vi "Run Contest.vi"() -> ()   [LabVIEW 2014]
uses:
  Participant.ctl
  Problem.ctl
  State Machine.ctl
  User Score Update.ctl
  Change Detect/Change Detect Int.vi
  Change Detect/Change Detect Boolean.vi
panel:
  in  "Update Ratings":bool
  in  "Early Finish":bool
  in  "Export Results":bool
  in  "Participant Names":string[](array[string])
  in  "Contest Length (hours)":dbl
  in  "Problem E Base Value":dbl=2500.0
  in  "Problem D Base Value":dbl=2000.0
  in  "Problem C Base Value":dbl=1500.0
  in  "Problem B Base Value":dbl=1000.0
  in  "Problem A Base Value":dbl=500.0
  in  "OK Button":bool
  in  "Problem":T1
  in  "Participant":string
  in  "At Time Remaining":dbl=3600.0
  out "Participant Status":T2[](array[typedef])
  in  "Participants":dbl
  in  "Contest Start":bool
  out "Time Remaining":u32
  out "Contest Indicator":bool
  out "Problem E Current Value":dbl
  out "Problem D Current Value":dbl
  out "Problem C Current Value":dbl
  out "Problem B Current Value":dbl
  out "Problem A Current Value":dbl
  # "You must export before starting a new Contest"
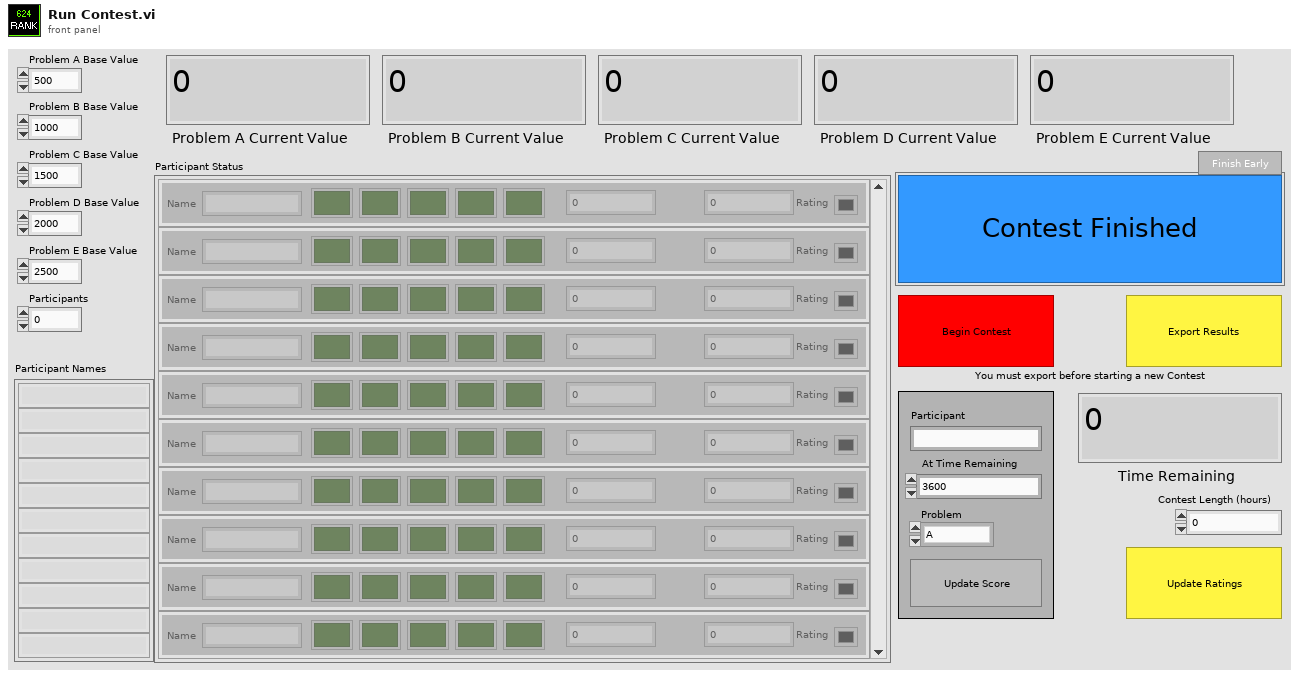
[diagram p1: front panel]
types:
  T1 = typedef "Problem.ctl" = enum16{"A", "B", "C", "D", "E"}
  T2 = typedef "Participant.ctl" = cluster{"Name":string, "A":bool, "Score":dbl, "B":bool, "C":bool, "D":bool, "E":bool, "Rating":dbl, "Color Box":u32}
  T3 = typedef "State Machine.ctl" = enum16{"Finish Contest", "Run Contest", "Begin Contest", "Wait for Start"}
  T4 = typedef "User Score Update.ctl" = cluster{"Score":dbl, "Name":string}
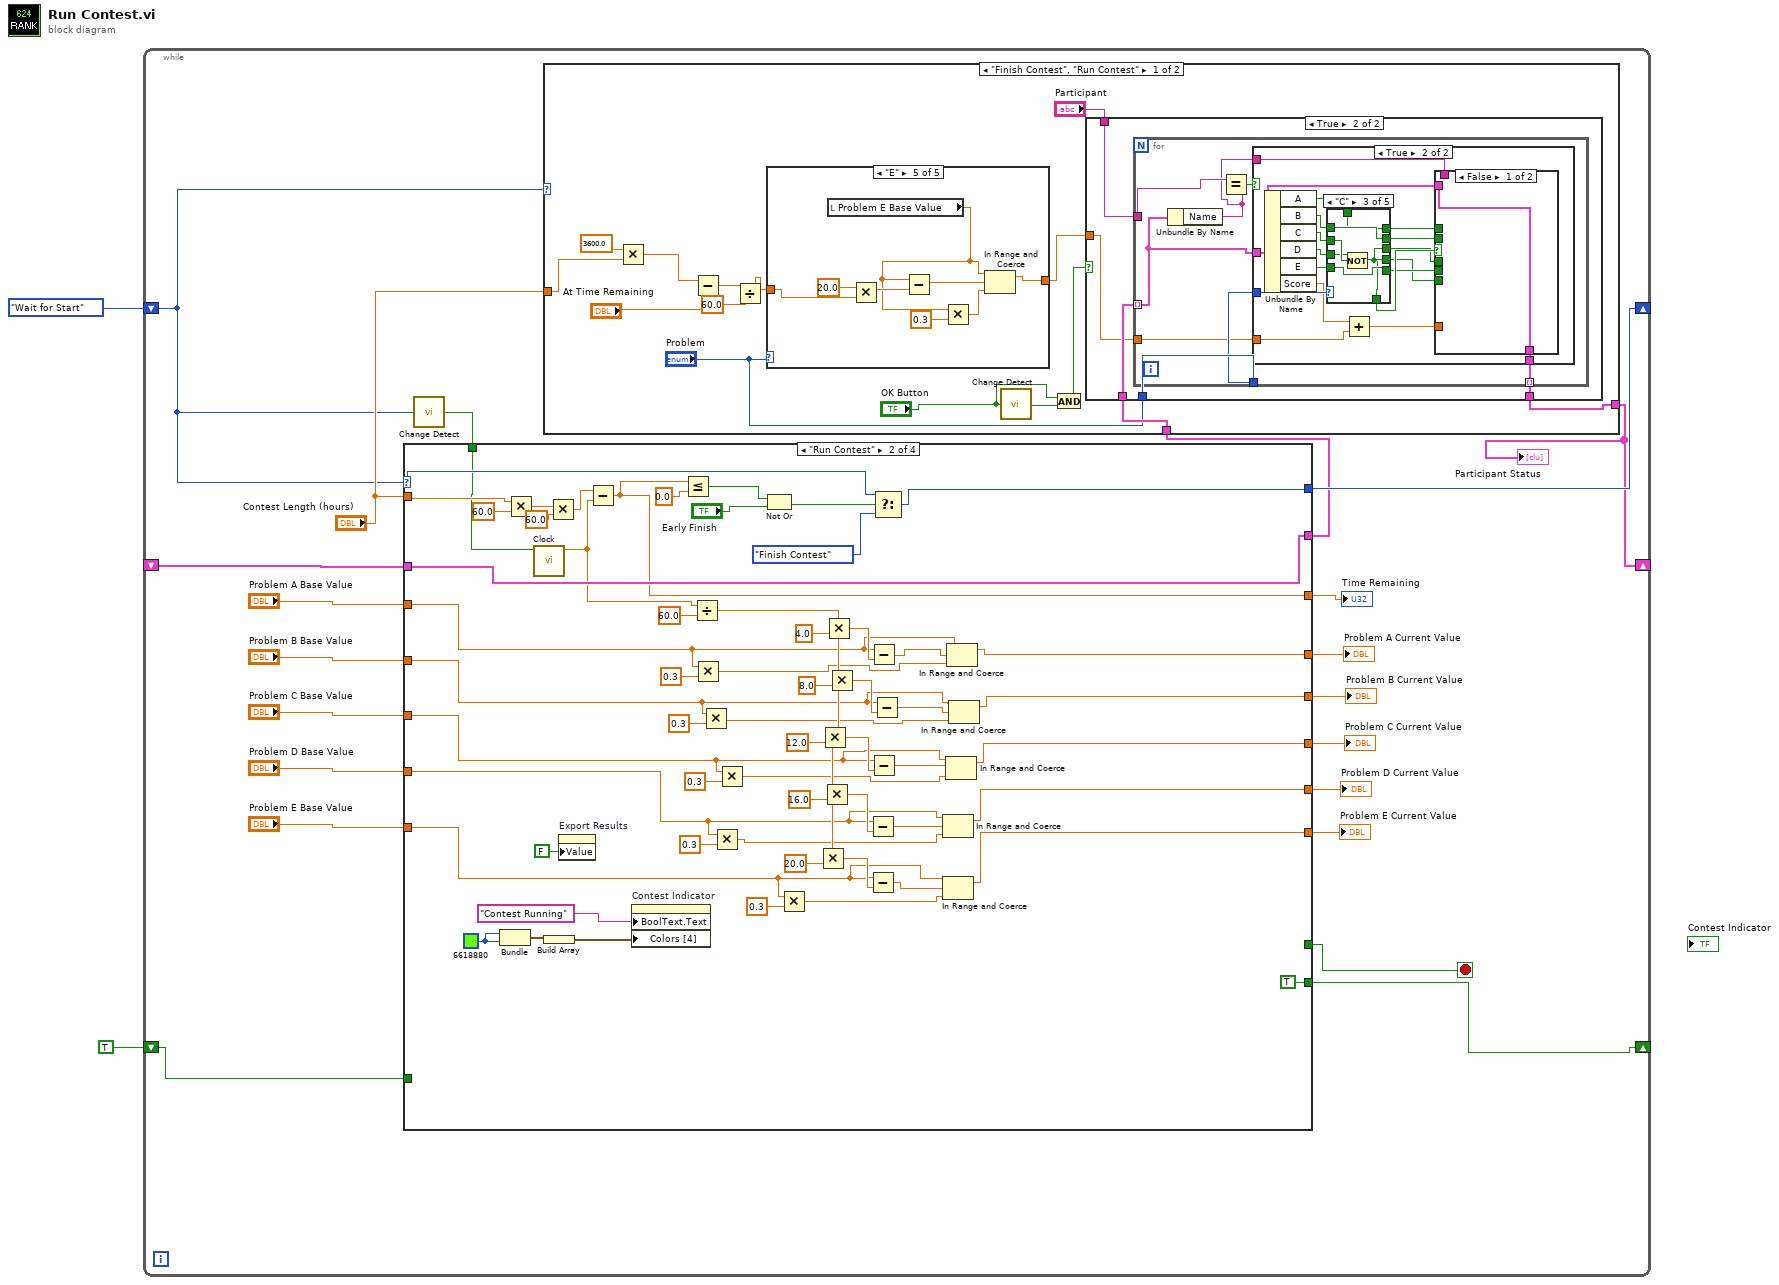
[diagram p0: block diagram]
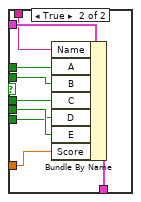
[diagram p4: hidden frame]
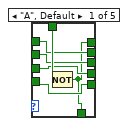
[diagram p5: hidden frame]
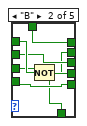
[diagram p6: hidden frame]
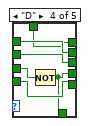
[diagram p7: hidden frame]
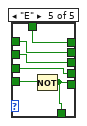
[diagram p8: hidden frame]
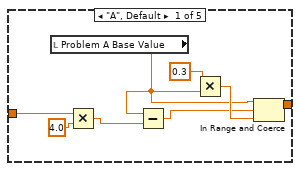
[diagram p9: hidden frame]
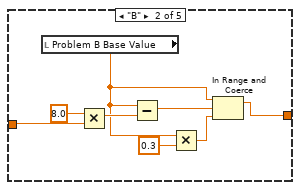
[diagram p10: hidden frame]
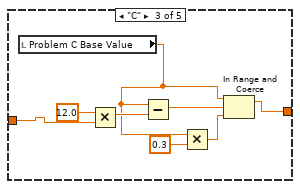
[diagram p11: hidden frame]
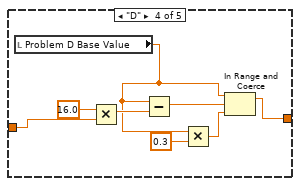
[diagram p12: hidden frame]
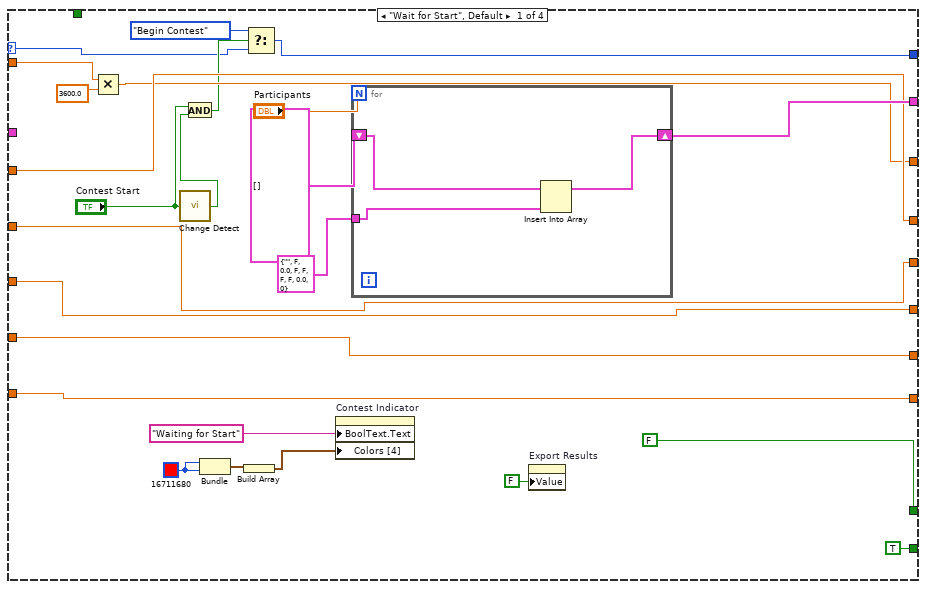
[diagram p14: hidden frame]
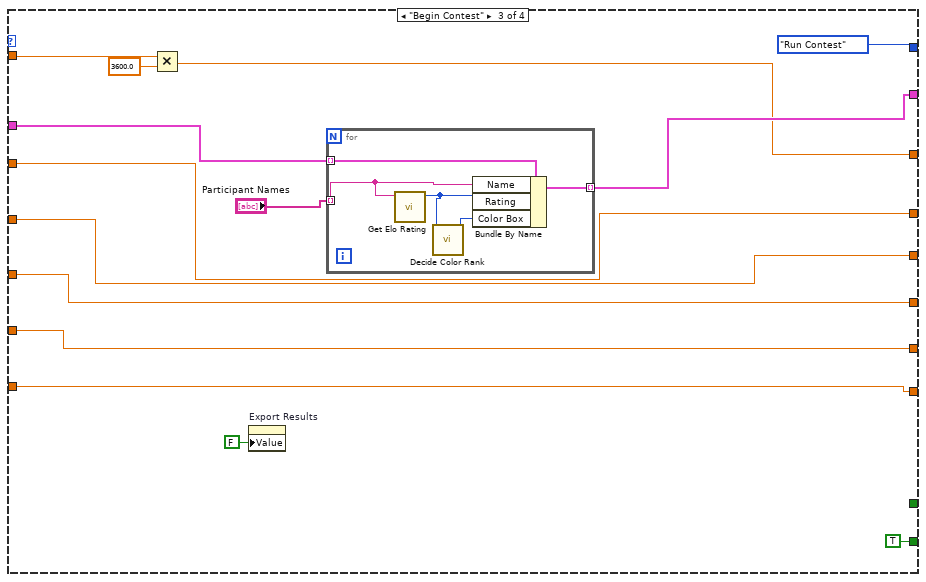
[diagram p15: hidden frame]
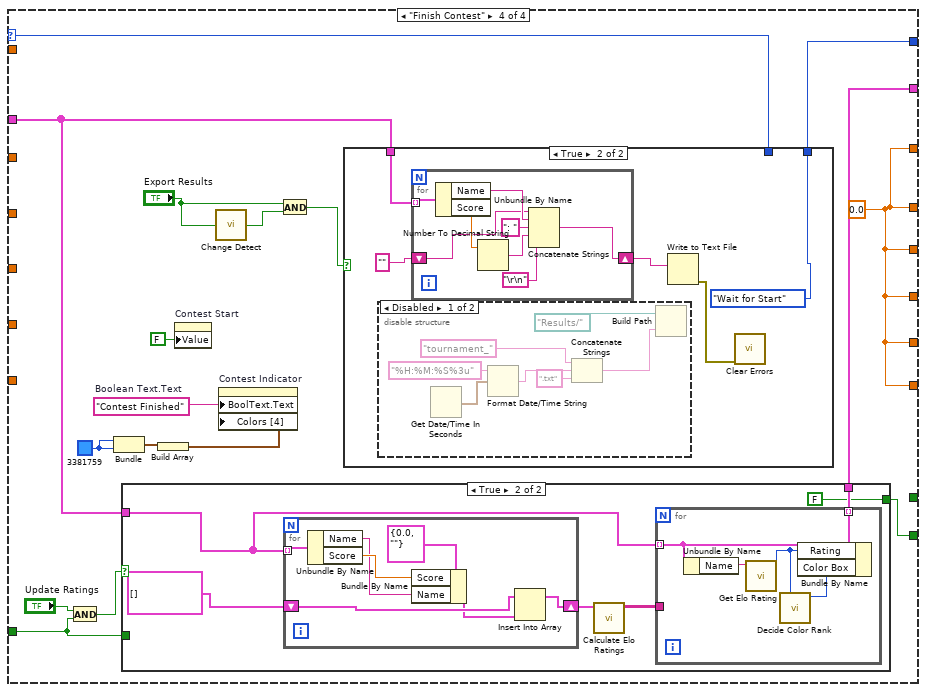
[diagram p16: hidden frame]
diagram:
  n1 = while {
    shift-right: [w6] -> _
    shift-left: _ -> [w22]
    shift-right: [w16] -> _
    shift-left: State_Machine."Wait for Start" -> [w5]
    shift-right: [w3] -> _
    shift-left: TRUE -> [w4]
    stop <- w23 stop-if-true
    n2 = call-poly "Change Detect.vi"("In"=w5) -> ("Changed?"=w9:bool)
    n3 = case shown="\"Run Contest\"" w5 {
      selector: w5 -> [w154 w228 _ w266]
      tunnel: [FALSE _ _ _] -> w23
      tunnel: [w172 w226 w250 w262] -> w7
      tunnel: w22 -> [_ w226 w251 w263]
      tunnel: "Problem A Base Value" -> [w163 w211 w248 _]
      tunnel: "Problem B Base Value" -> [w164 w203 w247 _]
      tunnel: "Problem C Base Value" -> [w165 w200 w246 _]
      tunnel: "Problem D Base Value" -> [w166 w195 w245 _]
      tunnel: "Problem E Base Value" -> [w167 w192 w244 _]
      tunnel: "Contest Length (hours)" -> [w162 w230 w243 _]
      tunnel: [w153 w227 State_Machine."Run Contest" w265] -> w16
      tunnel: [w163 w212 w248 w270] -> w15
      tunnel: [w164 w201 w247 w270] -> w14
      tunnel: [w165 w197 w246 w270] -> w13
      tunnel: [w166 w193 w245 w270] -> w12
      tunnel: [w167 w189 w244 w270] -> w11
      tunnel: [w160 w188 w241 w270] -> w10
      tunnel: w9 -> [_ w187 _ _]
      tunnel: w4 -> [_ _ _ w258]
      tunnel: [TRUE TRUE TRUE w259] -> w3
      frame "Wait for Start", Default {
        w170 = u32 16711680
        n4 = Multiply(x=w162, y=3600.0) -> (x*y=w160:dbl)
        n5 = call-poly "Change Detect.vi"("In"="Contest Start") -> ("Changed?"=w157:bool)
        n6 = And(x="Contest Start", y=w157) -> (x .and. y?=w156:bool)
        n7 = Bundle(w170, w170) -> (w169:cluster{u32, u32})  [unwired: 1 in]
        n8 = Build Array(w169) -> (w168:cluster{u32, u32}[])
        n9 = Select(t=State_Machine."Begin Contest", s=w156, f=w154) -> (s? t:f=w153:T3)
        n10 = property on="Contest Indicator" class="Bool (strict)"("BoolText.Text"="Waiting for Start" ("Boolean Text.Text"), "Colors [4]"=w168) -> ()  [unwired: 2 in, 2 out]
        n11 = for {
          N: "Participants" -> [_]
          shift-right: [w179] -> w172
          shift-left: T2[] [] ("array") -> [w178]
          tunnel: T2 {"Name"="", "A"=FALSE, "Score"=0.0, "B"=FALSE, "C"=FALSE, "D"=FALSE, "E"=FALSE, "Rating"=0.0, "Color Box"=0} ("Participant") -> [w177]
          n12 = Insert Into Array(array=w178, new element=w177) -> (w179:T2[])  [unwired: 1 in]
        }
        n13 = property on="Export Results" class="Bool (strict)"("Value"=FALSE ("Export Results")) -> ()  [unwired: 2 in, 2 out]
      }
      frame "Run Contest" {
        w237 = u32 6618880
        n14 = Bundle(w237, w237) -> (w236:cluster{u32, u32})  [unwired: 1 in]
        n15 = Multiply(x=w230, y=60.0) -> (x*y=w232:dbl)
        n16 = call "Clock.vi"("Reset?"=w187) -> ("Time Elapsed"=w186:dbl)  [unwired: 10 in]
        n17 = Build Array(w236) -> (w235:cluster{u32, u32}[])
        n18 = Multiply(x=w232, y=60.0) -> (x*y=w234:dbl)
        n19 = property on="Export Results" class="Bool (strict)"("Value"=FALSE ("Export Results")) -> ()  [unwired: 2 in, 2 out]
        n20 = Subtract(x=w234, y=w186) -> (x-y=w188:dbl)
        n21 = property on="Contest Indicator" class="Bool (strict)"("BoolText.Text"="Contest Running" ("Boolean Text.Text"), "Colors [4]"=w235) -> ()  [unwired: 2 in, 2 out]
        n22 = Less Or Equal?(x=w188, y=0.0) -> (x <= y?=w184:bool)
        n23 = Divide(x=w186, y=60.0) -> (x/y=w224:dbl)
        n24 = Multiply(x=w211, y=0.3) -> (x*y=w209:dbl)
        n25 = Multiply(x=w203, y=0.3) -> (x*y=w202:dbl)
        n26 = Multiply(x=w195, y=0.3) -> (x*y=w194:dbl)
        n27 = Multiply(x=w200, y=0.3) -> (x*y=w199:dbl)
        n28 = Not Or(1:"Early Finish", 2:w184) -> (0:w183:bool)
        n29 = Multiply(x=w192, y=0.3) -> (x*y=w191:dbl)
        n30 = Multiply(x=w224, y=20.0) -> (x*y=w214:dbl)
        n31 = Multiply(x=w224, y=12.0) -> (x*y=w216:dbl)
        n32 = Multiply(x=w224, y=16.0) -> (x*y=w215:dbl)
        n33 = Multiply(x=w224, y=4.0) -> (x*y=w218:dbl)
        n34 = Multiply(x=w224, y=8.0) -> (x*y=w217:dbl)
        n35 = Subtract(x=w195, y=w215) -> (x-y=w196:dbl)
        n36 = Subtract(x=w192, y=w214) -> (x-y=w190:dbl)
        n37 = Subtract(x=w211, y=w218) -> (x-y=w213:dbl)
        n38 = Subtract(x=w200, y=w216) -> (x-y=w198:dbl)
        n39 = Subtract(x=w203, y=w217) -> (x-y=w204:dbl)
        n40 = Select(t=w228, s=w183, f=State_Machine."Finish Contest") -> (s? t:f=w227:T3)
        n41 = In Range and Coerce(upper limit=w195, x=w196, lower limit=w194) -> (coerced(x)=w193:dbl)  [unwired: 1 out]
        n42 = In Range and Coerce(upper limit=w192, x=w190, lower limit=w191) -> (coerced(x)=w189:dbl)  [unwired: 1 out]
        n43 = In Range and Coerce(upper limit=w200, x=w198, lower limit=w199) -> (coerced(x)=w197:dbl)  [unwired: 1 out]
        n44 = In Range and Coerce(upper limit=w211, x=w213, lower limit=w209) -> (coerced(x)=w212:dbl)  [unwired: 1 out]
        n45 = In Range and Coerce(upper limit=w203, x=w204, lower limit=w202) -> (coerced(x)=w201:dbl)  [unwired: 1 out]
      }
      frame "Begin Contest" {
        n46 = Multiply(x=w243, y=3600.0) -> (x*y=w241:dbl)
        n47 = property on="Export Results" class="Bool (strict)"("Value"=FALSE ("Export Results")) -> ()  [unwired: 2 in, 2 out]
        n48 = for {
          tunnel: w251 -> [w257] mode=indexing
          tunnel: "Participant Names" -> [w255] mode=indexing
          tunnel: [w256] -> w250 mode=indexing
          n49 = call "Get Elo Rating.vi"("Name"=w255) -> ("Rating"=w254:i32)  [unwired: 10 in]
          n50 = call "Decide Color Rank.vi"("Numeric"=w254) -> ("Color Box"=w253:u32)  [unwired: 10 in]
          n51 = Bundle By Name(cluster=w257, "Name"=w255, "Rating"=w254, "Color Box"=w253) -> (w256:T2)
        }
      }
      frame "Finish Contest" {
        w270 = 0.0 ("Problem A Base Value")
        w273 = u32 3381759
        w271 = "Contest Finished"  # Boolean Text.Text
        n52 = And(x="Update Ratings", y=w258) -> (x .and. y?=w260:bool)
        n53 = Bundle(w273, w273) -> (w274:cluster{u32, u32})  [unwired: 1 in]
        n54 = case shown="True" w260 {
          tunnel: w263 -> [w276 w279]
          tunnel: [w276 w278] -> w262
          tunnel: [w275 FALSE] -> w259
          tunnel: w258 -> [w275 _]
          frame False {
          }
          frame True {
            n55 = for {
              tunnel: w279 -> [w294] mode=indexing
              shift-right: [w288] -> w281
              shift-left: T4[] [] ("Names") -> [w290]
              n56 = Unbundle By Name(w294) -> ("Name"=w291:string, "Score"=w292:dbl)
              n57 = Bundle By Name(cluster=T4 {"Score"=0.0, "Name"=""} ("Score Update"), "Score"=w292, "Name"=w291) -> (w289:T4)
              n58 = Insert Into Array(array=w290, new element=w289) -> (w288:T4[])  [unwired: 1 in]
            }
            n59 = call "Calculate Elo Ratings.vi"("Names"=w281) -> ("Rating 2D Array"=w280:string[][])  [unwired: 8 in, 2 out]
            n60 = for {
              tunnel: w280 -> [_]
              tunnel: w279 -> [w287] mode=indexing
              tunnel: [w285] -> w278 mode=indexing
              n61 = Unbundle By Name(w287) -> ("Name"=w286:string)
              n62 = call "Get Elo Rating.vi"("Name"=w286) -> ("Rating"=w284:i32)  [unwired: 10 in]
              n63 = call "Decide Color Rank.vi"("Numeric"=w284) -> ("Color Box"=w283:u32)  [unwired: 10 in]
              n64 = Bundle By Name(cluster=w287, "Rating"=w284, "Color Box"=w283) -> (w285:T2)
            }
          }
        }
        n65 = Build Array(w274) -> (w272:cluster{u32, u32}[])
        n66 = property on="Contest Start" class="Bool (strict)"("Value"=FALSE ("Contest Start")) -> ()  [unwired: 2 in, 2 out]
        n67 = call-poly "Change Detect.vi"("In"="Export Results") -> ("Changed?"=w269:bool)
        n68 = property on="Contest Indicator" class="Bool (strict)"("BoolText.Text"=w271, "Colors [4]"=w272) -> ()  [unwired: 2 in, 2 out]
        n69 = And(x="Export Results", y=w269) -> (x .and. y?=w267:bool)
        n70 = case shown="True" w267 {
          tunnel: w263 -> [_ w300]
          tunnel: w266 -> [w295 _]
          tunnel: [w295 State_Machine."Wait for Start" ("f")] -> w265
          frame False {
          }
          frame True {
            n71 = disable-structure shown="Disabled" {
              frame Disabled {
                n72 = Get Date/Time In Seconds() -> (seconds since 1Jan1904=w306:timestamp)
                n73 = Format Date/Time String(time format string (%c)="%H:%M:%S%3u", seconds (now)=w306) -> (date/time string=w303:string)  [unwired: 1 in]
                n74 = Concatenate Strings("tournament_", w303, ".txt" ("string")) -> (w301:string)
                n75 = Build Path(base path=path "Results/", name or relative path=w301) -> ()  [unwired: 1 out]
              }
              frame Enabled {
              }
            }
            n76 = for {
              tunnel: w300 -> [w315] mode=indexing
              shift-right: [w308] -> w298
              shift-left: "" -> [w310]
              n77 = Unbundle By Name(w315) -> ("Name"=w314:string, "Score"=w312:dbl)
              n78 = Number To Decimal String(number=w312) -> (decimal integer string=w311:string)  [unwired: 1 in]
              n79 = Concatenate Strings(w310, w314, ": " ("string"), w311, "\r\n") -> (w308:string)
            }
            n80 = Write to Text File(text=w298) -> (error out=w297:errorcluster)  [unwired: 3 in, 2 out]
            n81 = call <vilib>:"Clear Errors.vi"("error in (no error)"=w297) -> ()  [unwired: 5 in, 2 out]
          }
        }
      }
    }
    "Problem A Current Value" <- w15
    "Problem B Current Value" <- w14
    "Problem C Current Value" <- w13
    "Problem D Current Value" <- w12
    "Problem E Current Value" <- w11
    "Time Remaining" <- w10
    n82 = case shown="\"Finish Contest\", \"Run Contest\"" w5 {
      tunnel: "Contest Length (hours)" -> [w37 _]
      tunnel: w7 -> [w29 w151]
      tunnel: [w27 w151] -> w6
      frame "Finish Contest", "Run Contest" {
        n83 = Multiply(x=3600.0, y=w37) -> (x*y=w36:dbl)
        n84 = Subtract(x=w36, y="At Time Remaining") -> (x-y=w26:dbl)
        n85 = Divide(x=w26, y=60.0) -> (x/y=w25:dbl)
        n86 = case shown="\"E\"" "Problem" {
          tunnel: w25 -> [w117 w126 w129 w137 w145]
          tunnel: [w111 w119 w127 w135 w143] -> w31
          frame "A", Default {
            n87 = local read "Problem A Base Value"() -> (w113:dbl)
            n88 = Multiply(x=w117, y=4.0) -> (x*y=w115:dbl)
            n89 = Subtract(x=w113, y=w115) -> (x-y=w112:dbl)
            n90 = Multiply(x=0.3 ("y"), y=w113) -> (x*y=w114:dbl)
            n91 = In Range and Coerce(upper limit=w113, x=w112, lower limit=w114) -> (coerced(x)=w111:dbl)  [unwired: 1 out]
          }
          frame "B" {
            n92 = local read "Problem B Base Value"() -> (w120:dbl)
            n93 = Multiply(x=8.0, y=w126) -> (x*y=w124:dbl)
            n94 = Subtract(x=w120, y=w124) -> (x-y=w123:dbl)
            n95 = Multiply(x=w120, y=0.3) -> (x*y=w121:dbl)
            n96 = In Range and Coerce(upper limit=w120, x=w123, lower limit=w121) -> (coerced(x)=w119:dbl)  [unwired: 1 out]
          }
          frame "C" {
            n97 = local read "Problem C Base Value"() -> (w128:dbl)
            n98 = Multiply(x=12.0, y=w129) -> (x*y=w133:dbl)
            n99 = Subtract(x=w128, y=w133) -> (x-y=w132:dbl)
            n100 = Multiply(x=w128, y=0.3) -> (x*y=w130:dbl)
            n101 = In Range and Coerce(upper limit=w128, x=w132, lower limit=w130) -> (coerced(x)=w127:dbl)  [unwired: 1 out]
          }
          frame "D" {
            n102 = local read "Problem D Base Value"() -> (w136:dbl)
            n103 = Multiply(x=16.0, y=w137) -> (x*y=w139:dbl)
            n104 = Subtract(x=w136, y=w139) -> (x-y=w140:dbl)
            n105 = Multiply(x=w136, y=0.3) -> (x*y=w142:dbl)
            n106 = In Range and Coerce(upper limit=w136, x=w140, lower limit=w142) -> (coerced(x)=w135:dbl)  [unwired: 1 out]
          }
          frame "E" {
            n107 = local read "Problem E Base Value"() -> (w144:dbl)
            n108 = Multiply(x=20.0, y=w145) -> (x*y=w147:dbl)
            n109 = Subtract(x=w144, y=w147) -> (x-y=w148:dbl)
            n110 = Multiply(x=w144, y=0.3) -> (x*y=w150:dbl)
            n111 = In Range and Coerce(upper limit=w144, x=w148, lower limit=w150) -> (coerced(x)=w143:dbl)  [unwired: 1 out]
          }
        }
        n112 = call-poly "Change Detect.vi"("In"="OK Button") -> ("Changed?"=w34:bool)
        n113 = And(x="OK Button", y=w34) -> (x .and. y?=w32:bool)
        n114 = case shown="True" w32 {
          tunnel: w31 -> [_ w41]
          tunnel: "Participant" -> [_ w43]
          tunnel: w29 -> [w39 w44]
          tunnel: "Problem" -> [_ w42]
          tunnel: [w39 w40] -> w27
          frame False {
          }
          frame True {
            n115 = for {
              tunnel: w44 -> [w48] mode=indexing
              tunnel: w43 -> [w50]
              tunnel: w42 -> [w51]
              tunnel: w41 -> [w47]
              tunnel: [w45] -> w40 mode=indexing
              n116 = Unbundle By Name(w48) -> ("Name"=w46:string)
              n117 = Equal?(x=w50, y=w46) -> (x = y?=w49:bool)
              n118 = case shown="True" w49 {
                tunnel: w51 -> [_ w70]
                tunnel: w48 -> [w52 w64]
                tunnel: w47 -> [_ w62]
                tunnel: w46 -> [_ w60]
                tunnel: [w52 w53] -> w45
                frame False {
                }
                frame True {
                  n119 = Unbundle By Name(w64) -> ("A"=w69:bool, "B"=w68:bool, "C"=w67:bool, "D"=w66:bool, "E"=w65:bool, "Score"=w63:dbl)
                  n120 = case shown="\"C\"" w70 {
                    tunnel: w69 -> [w86 w91 w96 w100 w109]
                    tunnel: w68 -> [w85 w92 w97 w101 w108]
                    tunnel: w67 -> [w84 w90 w98 w102 w107]
                    tunnel: w66 -> [w83 w89 w95 w104 w106]
                    tunnel: w65 -> [w82 w88 w94 w103 w110]
                    tunnel: [w82 w88 w94 w103 w105] -> w58
                    tunnel: [w81 w91 w96 w100 w109] -> w54
                    tunnel: [w85 w87 w97 w101 w108] -> w55
                    tunnel: [w84 w90 w93 w102 w107] -> w56
                    tunnel: [w83 w89 w95 w99 w106] -> w57
                    tunnel: [w81 w87 w93 w99 w105] -> w59
                    frame "A", Default {
                      n121 = Not(x=w86) -> (.not. x?=w81:bool)
                    }
                    frame "B" {
                      n122 = Not(x=w92) -> (.not. x?=w87:bool)
                    }
                    frame "C" {
                      n123 = Not(x=w98) -> (.not. x?=w93:bool)
                    }
                    frame "D" {
                      n124 = Not(x=w104) -> (.not. x?=w99:bool)
                    }
                    frame "E" {
                      n125 = Not(x=w110) -> (.not. x?=w105:bool)
                    }
                  }
                  n126 = Add(x=w63, y=w62) -> (x+y=w61:dbl)
                  n127 = case shown="False" w59 {
                    tunnel: w64 -> [w71 w80]
                    tunnel: w61 -> [_ w78]
                    tunnel: w60 -> [_ w79]
                    tunnel: w58 -> [_ w77]
                    tunnel: w57 -> [_ w76]
                    tunnel: w56 -> [_ w75]
                    tunnel: w55 -> [_ w74]
                    tunnel: w54 -> [_ w73]
                    tunnel: [w71 w72] -> w53
                    frame False {
                    }
                    frame True {
                      n128 = Bundle By Name(cluster=w80, "Name"=w79, "A"=w73, "B"=w74, "C"=w75, "D"=w76, "E"=w77, "Score"=w78) -> (w72:T2)
                    }
                  }
                }
              }
            }
          }
        }
      }
      frame "Begin Contest", Default {
      }
    }
    "Participant Status" <- w6
  }
